vi "joystick+grsim.vi"() -> ()   [LabVIEW 2016]
uses:
  <vilib>/Utility/inputDevices.llb/closeJoystick.vi
panel:
  out "speed out":sgl[](array[numeric])
  out "16bit integer 3":i16
  out "16bit integer 2":i16
  out "16bit integer":i16
  out "appended array":u8[](array[numeric])
  out "error out 3":errorcluster
  in  "stop":bool
  in  "pos 1":i16=3468
  in  "pos 2":i16=3468
  in  "pos 3":i16=3468
  out "vel radial":u8[](array[numeric])
  out "vel normal":u8[](array[numeric])
  out "vel rotation":u8[](array[numeric])
  out "drible":u8
  # "vtan"
  # "vnorm"
  # "vang"
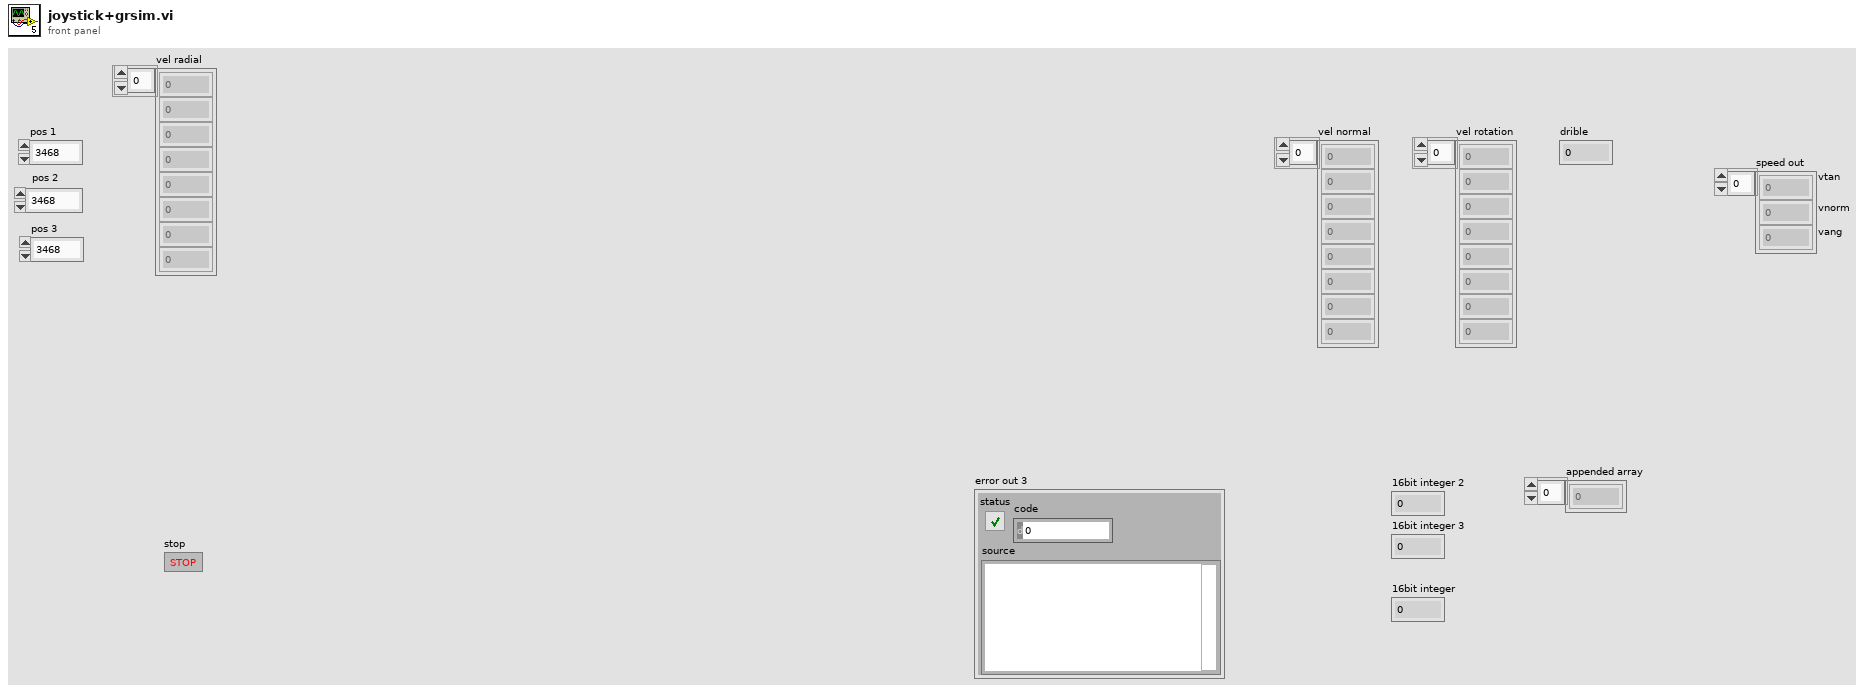
[diagram p1: front panel]
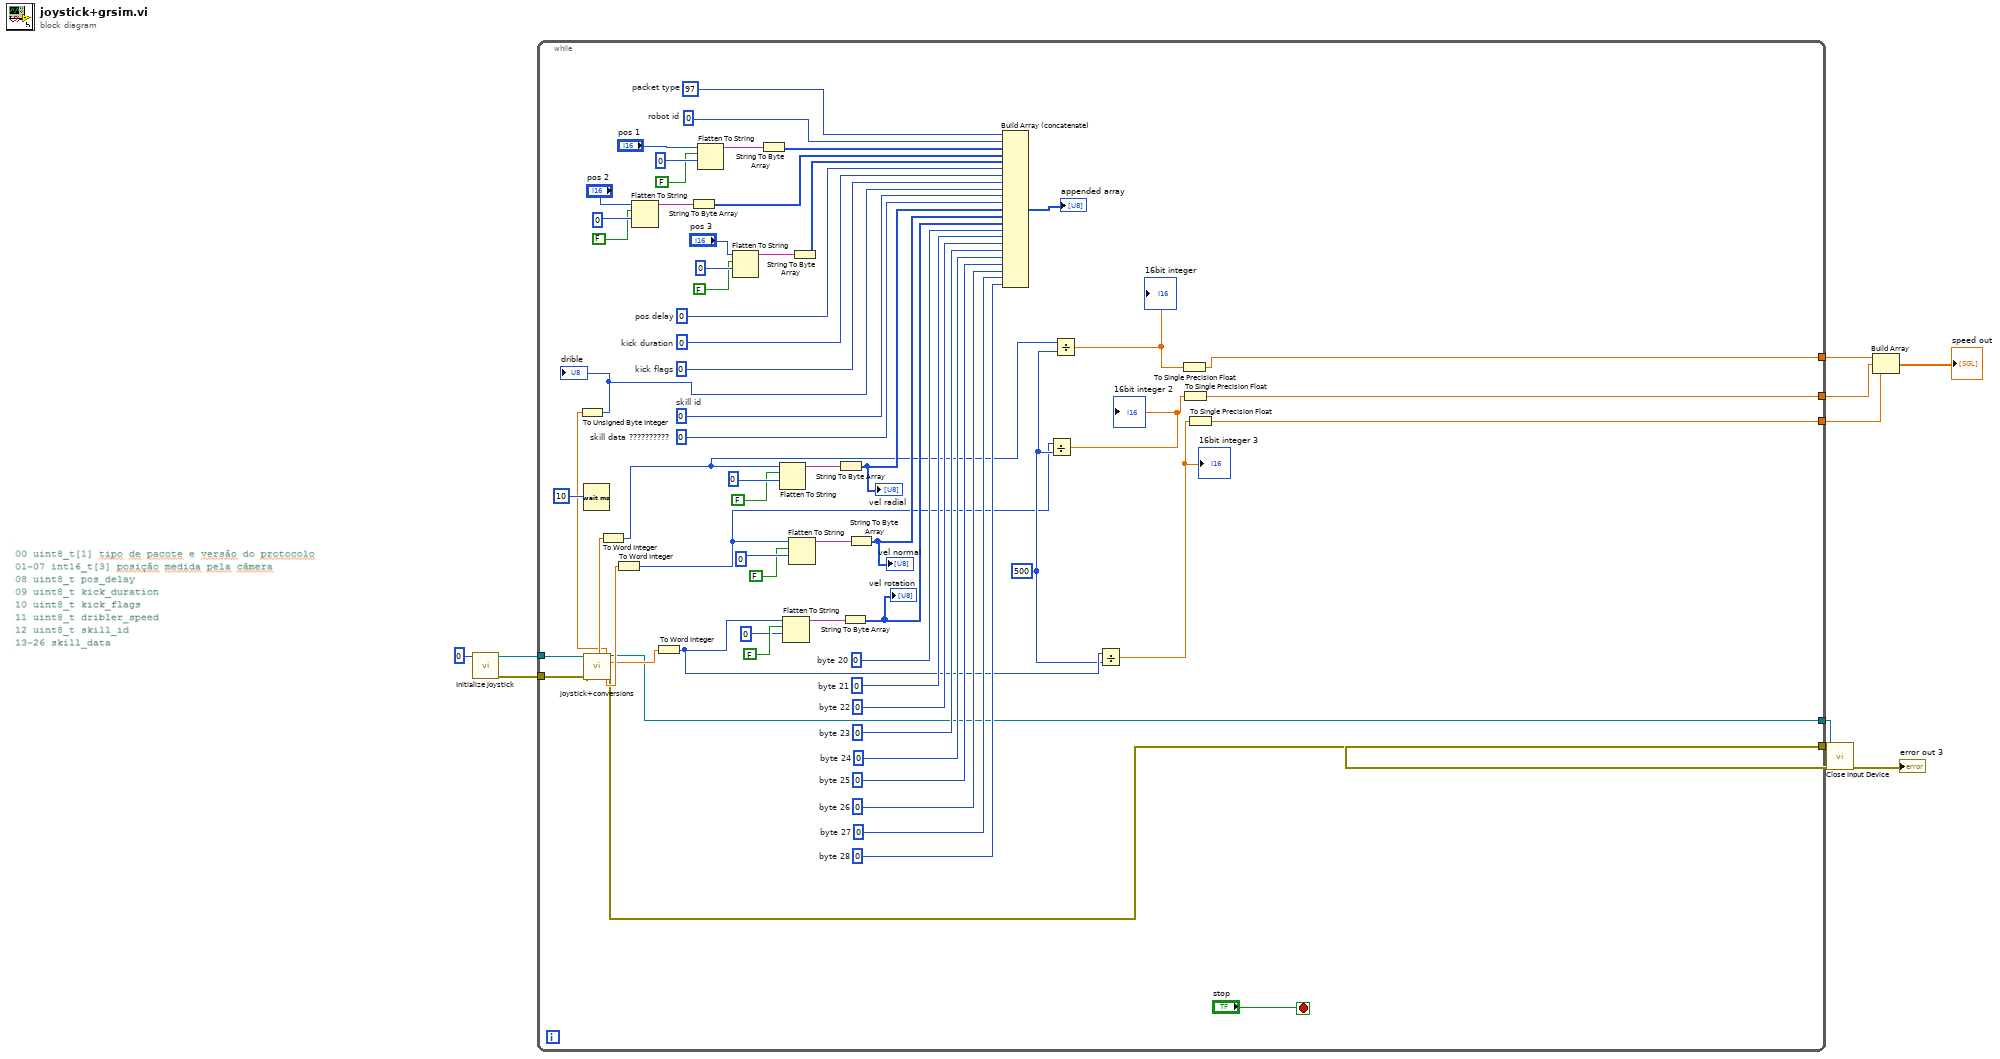
[diagram p0: block diagram]
diagram:
  n1 = call <vilib>:"Initialize Joystick.vi"("device index"=0) -> ("error out"=w8:errorcluster, "device ID"=w9:refnum<k1>)  [unwired: 9 in]
  n2 = while {
    tunnel: w9 -> [w32]
    tunnel: w8 -> [w31]
    tunnel: [w25] -> w6
    tunnel: [w24] -> w5
    tunnel: [w13] -> w4
    tunnel: [w12] -> w3
    tunnel: [w11] -> w2
    stop <- "stop" stop-if-true
    w18 = 500
    w74 = u8 0  # skill data ??????????
    w71 = u8 0  # byte 28
    w70 = u8 0  # byte 27
    w69 = u8 0  # byte 26
    w67 = u8 0  # byte 25
    w68 = u8 0  # byte 24
    w66 = u8 0  # byte 23
    w65 = u8 0  # byte 22
    w64 = u8 0  # byte 21
    w63 = u8 0  # byte 20
    w57 = u8 0  # skill id
    w62 = u8 0  # kick flags
    w56 = u8 0  # kick duration
    w55 = u8 0  # pos delay
    w60 = u8 0  # robot id
    w33 = u8 97  # packet type
    n3 = Wait (ms)(milliseconds to wait=u32 10) -> ()  [unwired: 1 out]
    n4 = call "joystick+conversions.vi"("Refnum in"=w32, "error in (no error)"=w31) -> ("v_radial"=w30:dbl, "drible"=w26:dbl, "v_normal"=w29:dbl, "Refnum out"=w24:refnum<k1>, "R*w"=w28:dbl, "error out"=w25:errorcluster)  [unwired: 9 in, 11 out]
    n5 = To Unsigned Byte Integer(number=w26) -> (unsigned 8bit integer=w27:u8)
    "drible" <- w27
    n6 = To Word Integer(number=w30) -> (16bit integer=w20:i16)
    n7 = To Word Integer(number=w29) -> (16bit integer=w16:i16)
    n8 = Flatten To String(anything="pos 2", prepend array or string size? (T)=FALSE, byte order (0:big-endian, network order)=u16 0) -> (data string=w41:string)  [unwired: 1 in, 2 out]
    n9 = To Word Integer(number=w28) -> (16bit integer=w19:i16)
    n10 = String To Byte Array(string=w41) -> (unsigned byte array=w61:u8[])
    n11 = Flatten To String(anything="pos 1", prepend array or string size? (T)=FALSE, byte order (0:big-endian, network order)=u16 0) -> (data string=w36:string)  [unwired: 1 in, 2 out]
    n12 = Flatten To String(anything="pos 3", prepend array or string size? (T)=FALSE, byte order (0:big-endian, network order)=u16 0) -> (data string=w45:string)  [unwired: 1 in, 2 out]
    n13 = String To Byte Array(string=w36) -> (unsigned byte array=w37:u8[])
    n14 = Flatten To String(anything=w20, prepend array or string size? (T)=FALSE, byte order (0:big-endian, network order)=u16 0) -> (data string=w50:string)  [unwired: 1 in, 2 out]
    n15 = Flatten To String(anything=w19, prepend array or string size? (T)=FALSE, byte order (0:big-endian, network order)=u16 0) -> (data string=w54:string)  [unwired: 1 in, 2 out]
    n16 = Flatten To String(anything=w16, prepend array or string size? (T)=FALSE, byte order (0:big-endian, network order)=u16 0) -> (data string=w53:string)  [unwired: 1 in, 2 out]
    n17 = String To Byte Array(string=w45) -> (unsigned byte array=w47:u8[])
    n18 = String To Byte Array(string=w50) -> (unsigned byte array=w72:u8[])
    "vel radial" <- w72
    n19 = String To Byte Array(string=w54) -> (unsigned byte array=w73:u8[])
    "vel rotation" <- w73
    n20 = String To Byte Array(string=w53) -> (unsigned byte array=w21:u8[])
    "vel normal" <- w21
    n21 = Build Array (concatenate)(w33, w60, w37, w61, w47, w55, w56, w62, w27, w57, w74, w72, w21, w73, w63, w64, w65, w66, w68, w67, w69, w70, w71) -> (→"appended array":u8[])
    n22 = Divide(x=w16, y=w18) -> (x/y=w15:dbl)
    "16bit integer 2" <- w15
    n23 = Divide(x=w20, y=w18) -> (x/y=w17:dbl)
    "16bit integer" <- w17
    n24 = Divide(x=w19, y=w18) -> (x/y=w14:dbl)
    "16bit integer 3" <- w14
    n25 = To Single Precision Float(number=w17) -> (single precision float=w13:sgl)
    n26 = To Single Precision Float(number=w15) -> (single precision float=w12:sgl)
    n27 = To Single Precision Float(number=w14) -> (single precision float=w11:sgl)
  }
  n28 = call-poly <vilib>:"Close Input Device.vi"("error in (no error)"=w6, "device ID"=w5) -> ("error out"=→"error out 3":errorcluster)  [unwired: 8 in]
  n29 = Build Array(w4, w3, w2) -> (→"speed out":sgl[])
